vi "Configure Waveform Modulation Type.vi"(8 "error in (no error)":errorcluster, 9 "Modulation Type (0: Amplitude Modulation)":i32(ring) items=["Amplitude Modulation", "Frequency Modulation", "Frequency-Shift Keying Modulation"], 10 "Waveform Generator Number (1: Waveform Generator 1)":i32(ring)=1 items=["Waveform Generator 1"=1], 11 "VISA resource name":refnum<visa-resource-name>) -> (0 "error out":errorcluster, 3 "VISA resource name out":refnum<visa-resource-name>)   [LabVIEW 2016, in "Agilent 2000 3000 X-Series.lvlib"]
doc: "Selects the modulation type."
uses:
  Agilent 2000 3000 X-Series.lvlib
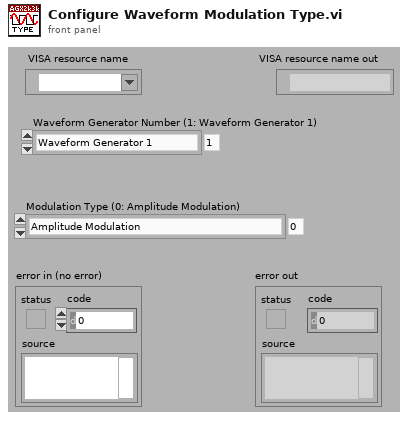
[diagram p1: front panel]
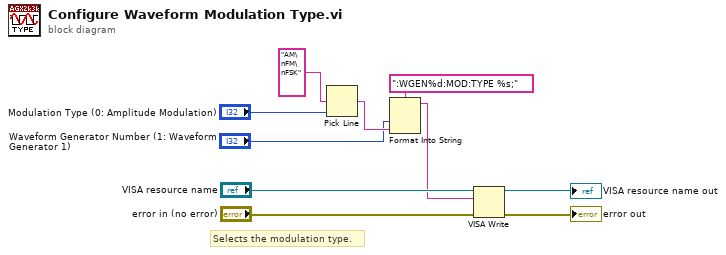
[diagram p0: block diagram]
diagram:
  # "Selects the modulation type."
  n1 = Pick Line(multi-line string="AM\nFM\nFSK", line index="Modulation Type (0: Amplitude Modulation)") -> (output string=w4:string)  [unwired: 1 out]
  n2 = Format Into String(format string=":WGEN%d:MOD:TYPE %s;", "Waveform Generator Number (1: Waveform Generator 1)", w4) -> (resulting string=w1:string)  [unwired: 2 in, 1 out]
  n3 = VISA Write(VISA resource name="VISA resource name", write buffer=w1, error in (no error)="error in (no error)") -> (VISA resource name out=→"VISA resource name out":refnum<visa-resource-name>, error out=→"error out":errorcluster)  [unwired: 1 out]
